vi "Reconstruct.vi"(8 "error in (no error)":errorcluster, 11 "Model Panel Logic in":refnum<class "Model Panel Logic Nested Window.lvclass">) -> (0 "error out":errorcluster, 3 "Model Panel Logic out":refnum<class "Model Panel Logic Nested Window.lvclass">)   [LabVIEW 2020, in "Form Model.lvlib" / "Model Panel Logic Nested Window.lvclass"]
uses:
  Model Panel Logic Nested Window.lvclass
  Model Panel Logic Nested Window.lvclass/Model Panel Logic Nested Window.ctl
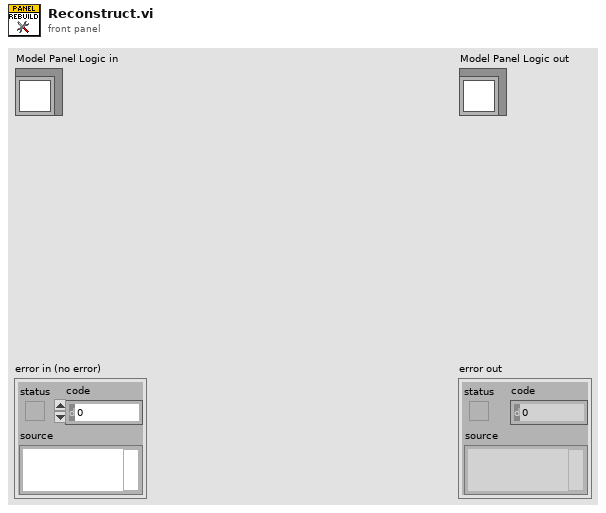
[diagram p1: front panel]
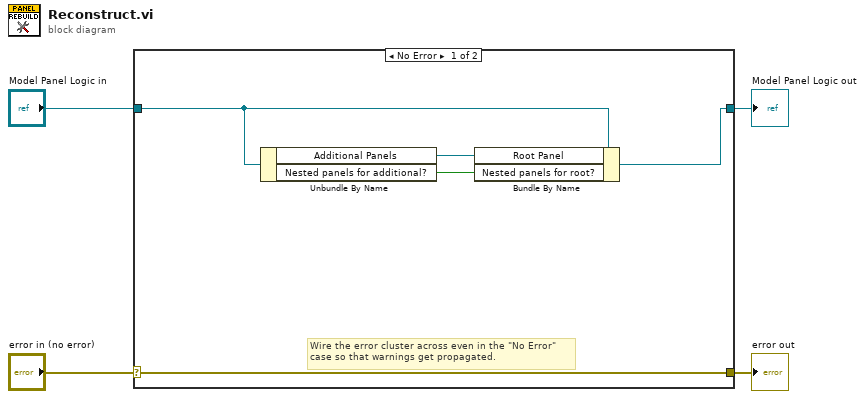
[diagram p0: block diagram]
diagram:
  n1 = case shown="No Error" "error in (no error)" {
    selector: "error in (no error)" -> [w9 w11]
    tunnel: [w9 w11] -> w3
    tunnel: [w7 w10] -> w1
    tunnel: "Model Panel Logic in" -> [w8 w10]
    frame No Error {
      # "Wire the error cluster across even in the \"No Error\"\ncase so that warnings get propagated."
      n2 = Unbundle By Name(w8) -> ("Additional Panels"=w6:refnum<class "Panel.lvclass">, "Nested panels for additional?"=w5:bool)
      n3 = Bundle By Name(cluster=w8, "Root Panel"=w6, "Nested panels for root?"=w5) -> (w7:refnum<class "Model Panel Logic Nested Window.lvclass">)
    }
    frame Error {
    }
  }
  "error out" <- w3
  "Model Panel Logic out" <- w1
